vi "PWM_CTR.vi"(10 "SIG_IN":bool) -> (1 "LOW CTR":u32, 2 "HIGH CTR":u32)   [LabVIEW 2013]
panel:
  # "this VI computes the HIGH and LOW time of the input signal\nit should be used in a SCTL in order to save resources and operate as fast as possible. Furthermore the RT-VIs rely on this VI to be placed in a SCTL, in order to measure the period in seconds\nThe HIGH CTR and LOW CTR can be used to measure the duty cycle of a PWM and its period! (We do that on the RT-side)"
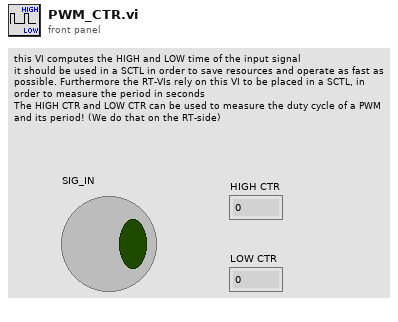
[diagram p1: front panel]
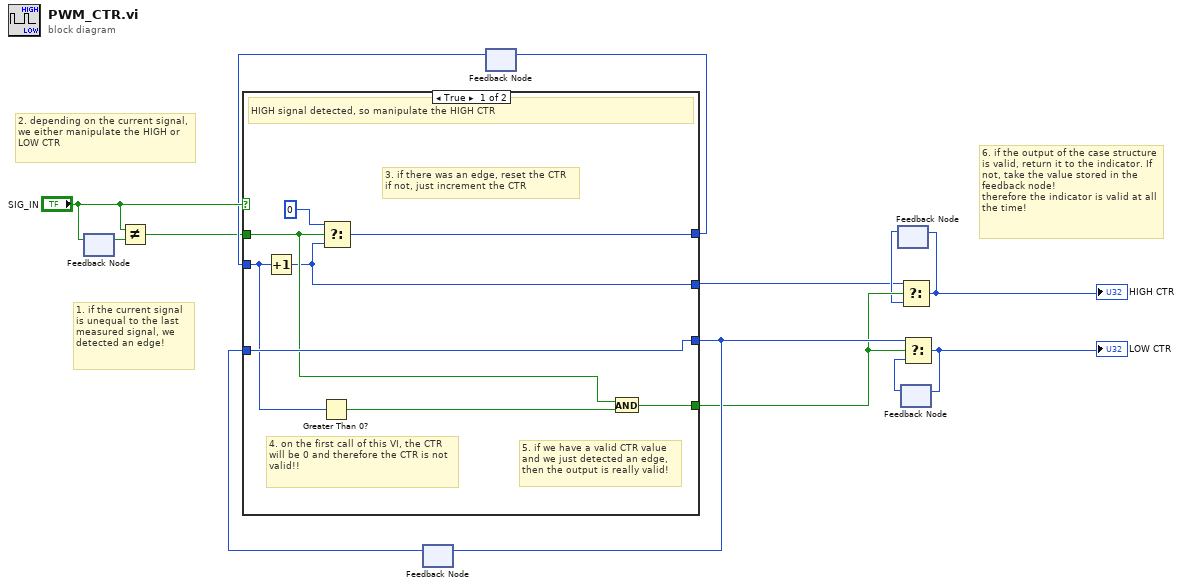
[diagram p0: block diagram]
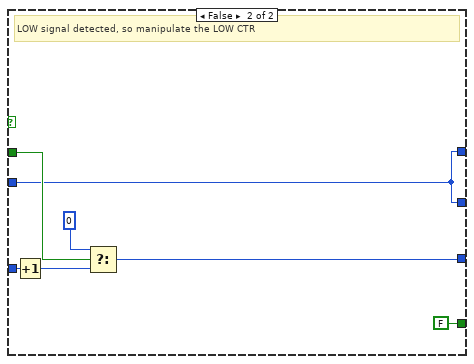
[diagram p2: hidden frame]
diagram:
  # "6. if the output of the case structure is valid, return it to the indicator. If not, take the value stored in the feedback node!\ntherefore the indicator is valid at all the time!"
  # "2. depending on the current signal, we either manipulate the HIGH or LOW CTR"
  # "1. if the current signal is unequal to the last measured signal, we detected an edge!"
  n1 = feedback #1() -> (w13:bool)  [unwired: 1 in]
  n2 = feedback-in #1("SIG_IN") -> ()
  n3 = Not Equal?(x="SIG_IN", y=w13) -> (x != y?=w9:bool)
  n4 = feedback #2() -> (w10:u32)  [unwired: 1 in]
  n5 = feedback #3() -> (w11:u32)  [unwired: 1 in]
  n6 = case shown="True" "SIG_IN" {
    tunnel: w9 -> [w18 w28]
    tunnel: w11 -> [w15 w22]
    tunnel: [w20 w22] -> w8
    tunnel: [w19 w25] -> w7
    tunnel: w10 -> [w19 w24]
    tunnel: [w16 FALSE] -> w6
    tunnel: [w14 w22] -> w1
    frame True {
      # "5. if we have a valid CTR value\nand we just detected an edge,\nthen the output is really valid!"
      # "4. on the first call of this VI, the CTR will be 0 and therefore the CTR is not valid!!"
      # "3. if there was an edge, reset the CTR\nif not, just increment the CTR"
      # "HIGH signal detected, so manipulate the HIGH CTR"
      n7 = Increment(x=w15) -> (x+1=w14:u32)
      n8 = Greater Than 0?(x=w15) -> (x > 0?=w17:bool)
      n9 = Select(t=u32 0 ("f"), s=w18, f=w14) -> (s? t:f=w20:u32)
      n10 = And(x=w18, y=w17) -> (x .and. y?=w16:bool)
    }
    frame False {
      # "LOW signal detected, so manipulate the LOW CTR"
      n11 = Increment(x=w24) -> (x+1=w26:u32)
      n12 = Select(t=u32 0 ("f"), s=w28, f=w26) -> (s? t:f=w25:u32)
    }
  }
  n13 = feedback-in #2(w7) -> ()
  n14 = feedback-in #3(w8) -> ()
  n15 = feedback #4() -> (w2:u32)  [unwired: 1 in]
  n16 = Select(t=w1, s=w6, f=w2) -> (s? t:f=w3:u32)
  "HIGH CTR" <- w3
  n17 = feedback-in #4(w3) -> ()
  n18 = feedback #5() -> (w4:u32)  [unwired: 1 in]
  n19 = Select(t=w7, s=w6, f=w4) -> (s? t:f=w5:u32)
  "LOW CTR" <- w5
  n20 = feedback-in #5(w5) -> ()
